vi "ExampleARGBImageData.vi"(8 "error in (no error)":errorcluster, 11 "Image Size":T3={"Width"=3, "Height"=2}) -> (0 "error out":errorcluster, 3 "Data Value Reference out":T1, 5 "ARGB Array Data":u32[][](array[numeric]), 7 "ARGB Pixmap Data":T2)   [LabVIEW 2020, in "g_ar_toolkit.test.lvlib" / "Image.lvclass"]
uses:
  Image.lvclass
  g_ar_toolkit.common/Image Size (Integer).ctl
  <vilib>/picture/picture.llb/imagedata.ctl
  g_ar_toolkit.image/ARGB Image.ctl
  g_ar_toolkit.image/New Image (ARGB).vi
  g_ar_toolkit.image/Copy Array to Image (ARGB).vi
  g_ar_toolkit.image/New Image (ARGB).vi/3321fa97-f432-4e1e-8db9-a0df79aed21b.vi
  g_ar_toolkit.image/ARGB Colour to U32 Pixel Value.vi
  g_ar_toolkit.common/Module Path.vi
  <vilib>/Utility/error.llb/Error Cluster From Error Code.vi
  Image.lvclass/Image.ctl
  g_ar_toolkit.image/g_ar_toolkit.image.lvlib
  g_ar_toolkit.common/g_ar_toolkit.common.lvlib
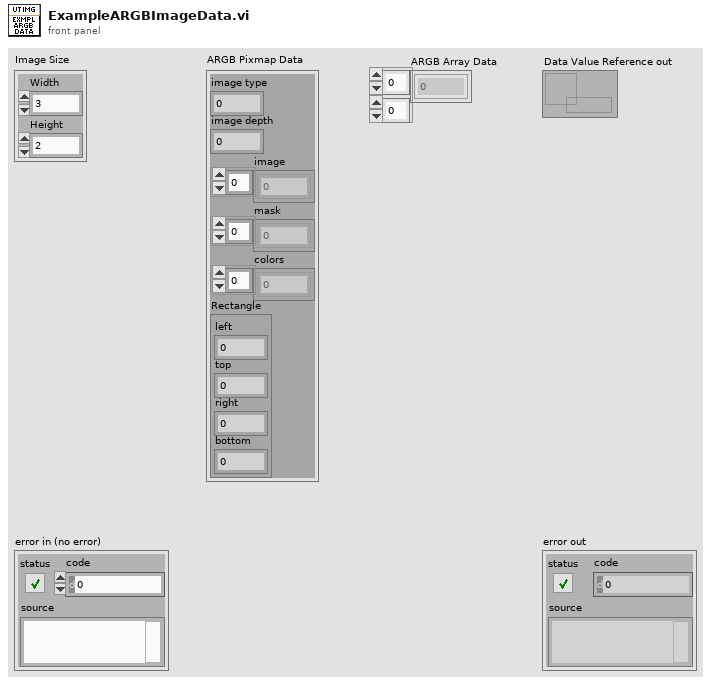
[diagram p1: front panel]
types:
  T1 = typedef "g_ar_toolkit.image.lvlib/ARGB Image.ctl" = refnum<data-value>
  T2 = typedef "imagedata.ctl" = cluster{"image type":i32, "image depth":i32, "image":u8[], "mask":u8[], "colors":u32[], "Rectangle":cluster{"left":i16, "top":i16, "right":i16, "bottom":i16}}
  T3 = typedef "g_ar_toolkit.common.lvlib/Image Size (Integer).ctl" = cluster{"Width":u16, "Height":u16}
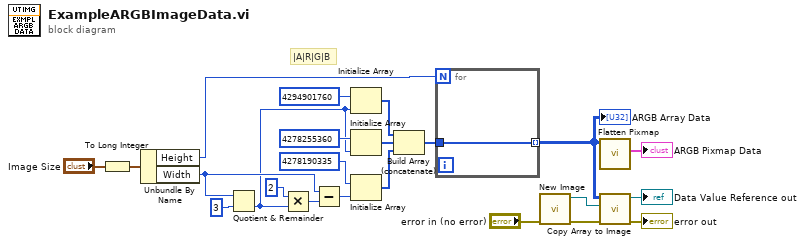
[diagram p0: block diagram]
diagram:
  # "|A|R|G|B"
  n1 = To Long Integer(number="Image Size") -> (32bit integer=w19:cluster{"Width":i32, "Height":i32})
  n2 = Unbundle By Name(w19) -> ("Height"=w8:i32, "Width"=w18:i32)
  n3 = Quotient & Remainder(x=w18, y=3) -> (floor(x/y)=w17:i32)  [unwired: 1 out]
  n4 = Multiply(x=2, y=w17) -> (x*y=w15:i32)
  n5 = Subtract(x=w18, y=w15) -> (x-y=w13:i32)
  n6 = Initialize Array(u32 4294901760, w17) -> (w12:u32[])
  n7 = Initialize Array(u32 4278255360, w17) -> (w11:u32[])
  n8 = Initialize Array(u32 4278190335, w13) -> (w10:u32[])
  n9 = Build Array (concatenate)(w12, w11, w10) -> (w9:u32[])
  n10 = for {
    N: w8 -> [_]
    tunnel: w9 -> [w24]
    tunnel: [w24] -> w1 mode=indexing
  }
  "ARGB Array Data" <- w1
  n11 = call-poly "New Image.vi"("error in (no error)"="error in (no error)") -> ("error out"=w5:errorcluster, "New ARGB Image"=w2:T1)  [unwired: 9 in]
  n12 = call <vilib>:"Flatten Pixmap.vi"("24-bit pixmap"=w1) -> ("image data"=→"ARGB Pixmap Data":T2)  [unwired: 10 in]
  n13 = call-poly "Copy Array to Image.vi"("error in (no error)"=w5, "ARGB Image Destination"=w2, "U32 ARBG Data"=w1) -> ("error out"=→"error out":errorcluster, "ARGB Image Destination (Duplicate)"=→"Data Value Reference out":T1)  [unwired: 7 in]
